vi "Detect Freeze.vi"(8 "error in (no error)":errorcluster, 11 "Running image Index":i32) -> (0 "error out":errorcluster)   [LabVIEW 2013]
doc: "Use this template to build a VI to use as a subVI."
uses:
  DB/DbEnum.ctl
  TypeDef/GreyLevelData.ctl
  DB/DisplayGFVEnum.ctl
  DB/DisplayDB.ctl
  <vilib>/vision/Image Controls.llb/IMAQ Image.ctl
  DB/ConfDB.ctl
  DB/ConfEnum.ctl
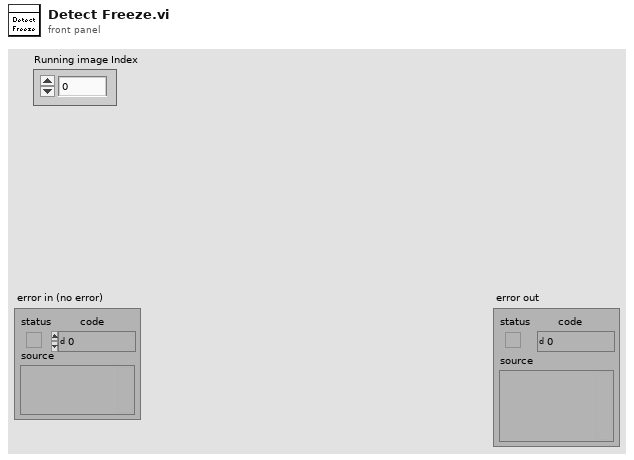
[diagram p1: front panel]
types:
  T1 = typedef "ConfEnum.ctl" = enum16{"Init", "GetConfDB", "Configure DB"}
  T2 = typedef "ConfDB.ctl" = cluster{"NumberOfImages":i32, "NoImages2SaveAroundFreeze":i32, "Path":path, "NameOfPartialFile":string, "StartIndex":i32, "NumberOfStdTol":i32, "Detla t (sec)":i32, "Number of images for baseline":i32, "Temperature File Name":string, "Score":dbl, "Index number of Files":i32[], "End Index":i32}
  T3 = cluster{"ImageIndexArray":u32[], "GreyLevelInBoundingBox":dbl[][], "GLDifference":dbl[][]}
  T4 = typedef "DbEnum.ctl" = enum16{"Init", "Insert Detection Result Data", "Insert Grey Level Result", "Insert Baseline Results", "Insert Freeze Analysis Results", "GetDropDB", "GetGreyLevelAndDiff", "GetGreyLevelatIndexTime", "GetDropletsBoundingBox"}
  T5 = typedef "DisplayDB.ctl" = cluster{"Image Ref":T6}
  T6 = typedef "IMAQ Image.ctl" = refnum<image>
  T7 = typedef "DisplayGFVEnum.ctl" = enum16{"Update Display", "Get Image Ref", "Insert Image Ref to Display", "Init Display"}
  T8 = typedef "GreyLevelData.ctl" = cluster{"Grey Level":dbl[], "Grey level diff":dbl[], "ImageIndex":u32, "Drop Index":u32}
  T9 = typedef "FreezePointData.ctl" = cluster{"Freeze YesNo":cluster{"Freeze Grey Diff value":dbl, "Freeze Index":u32, "Freeze Point Found":bool}[], "Rel Time":u32[]}
  T10 = cluster{"DropletBaseline":dbl[], "DropletBaselineSTD":dbl[]}
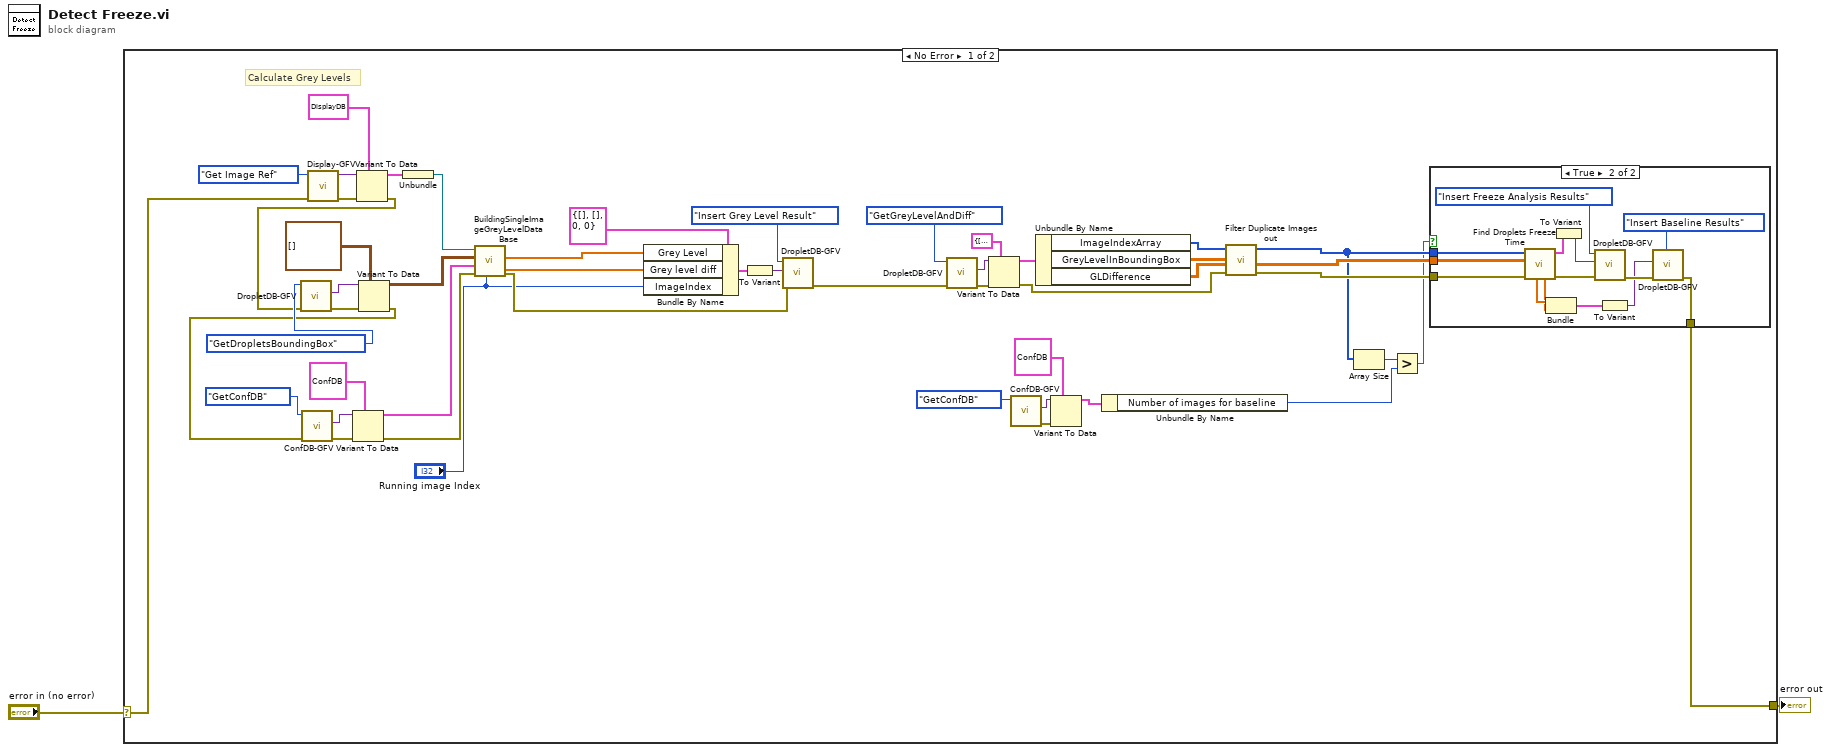
[diagram p0: block diagram]
diagram:
  n1 = case shown="No Error" "error in (no error)" {
    selector: "error in (no error)" -> [w33 w68]
    tunnel: [w12 w68] -> w1
    frame No Error {
      # "Calculate Grey Levels"
      n2 = call "Display-GFV.vi"("error in (no error)"=w33, 11:DisplayGFVEnum."Get Image Ref") -> ("error out"=w49:errorcluster, "Data out"=w48:variant)  [unwired: 7 in, 1 out]
      n3 = Variant To Data(error in=w49, type=T5 {"Image Ref"=refnum} ("Display Cluster"), Variant=w48) -> (data=w50:T5, error out=w32:errorcluster)
      n4 = call "DropletDB-GFV.vi"("error in (no error)"=w32, "Command In"=DbEnum."GetDropletsBoundingBox") -> ("error out"=w39:errorcluster, "Data out"=w40:variant)  [unwired: 8 in]
      n5 = Variant To Data(error in=w39, type=cluster{"x":sgl, "y":sgl}[][] [] ("Bounding Box"), Variant=w40) -> (data=w52:cluster{"x":sgl, "y":sgl}[][], error out=w31:errorcluster)
      n6 = call "ConfDB-GFV.vi"("error in (no error)"=w31, "Command In"=ConfEnum."GetConfDB") -> ("error out"=w35:errorcluster, "Data out"=w36:variant)  [unwired: 8 in]
      n7 = Variant To Data(error in=w35, type=T2 {"NumberOfImages"=0, "NoImages2SaveAroundFreeze"=0, "Path"=path "", "NameOfPartialFile"="", "StartIndex"=0, "NumberOfStdTol"=0, "Detla t (sec)"=0, "Number of images for baseline"=0, "Temperature File Name"="", "Score"=0.0, "Index number of Files"=[], "End Index"=0} ("ConfDB"), Variant=w36) -> (data=w26:T2, error out=w30:errorcluster)
      n8 = Unbundle(w50) -> ("Image Ref"=w51:T6)
      n9 = call "BuildingSingleImageGreyLevelDataBase.vi"("Running Index"="Running image Index", "error in (no error)"=w30, "ConfDB"=w26, "Droplet Bounding Box"=w52, "Image Ref In"=w51) -> ("error out"=w27:errorcluster, "Difference in Grey Level"=w28:dbl[], "GreyLevelArray"=w29:dbl[])  [unwired: 4 in]
      n10 = Bundle By Name(cluster=T8 {"Grey Level"=[], "Grey level diff"=[], "ImageIndex"=0, "Drop Index"=0} ("Cluster"), "Grey Level"=w29, "Grey level diff"=w28, "ImageIndex"="Running image Index") -> (w44:T8)
      n11 = To Variant(anything=w44) -> (Variant=w43:variant)
      n12 = call "DropletDB-GFV.vi"("error in (no error)"=w27, "Data in"=w43, "Command In"=DbEnum."Insert Grey Level Result") -> ("error out"=w23:errorcluster)  [unwired: 7 in, 1 out]
      n13 = call "DropletDB-GFV.vi"("error in (no error)"=w23, "Command In"=DbEnum."GetGreyLevelAndDiff") -> ("error out"=w22:errorcluster, "Data out"=w21:variant)  [unwired: 8 in]
      n14 = Variant To Data(error in=w22, type=T3 {"ImageIndexArray"=[], "GreyLevelInBoundingBox"=[], "GLDifference"=[]} ("output cluster"), Variant=w21) -> (data=w19:T3, error out=w15:errorcluster)
      n15 = call "ConfDB-GFV.vi"("Command In"=ConfEnum."GetConfDB") -> ("error out"=w7:errorcluster, "Data out"=w8:variant)  [unwired: 9 in]
      n16 = Unbundle By Name(w19) -> ("ImageIndexArray"=w18:u32[], "GreyLevelInBoundingBox"=w17:dbl[][], "GLDifference"=w16:dbl[][])
      n17 = Variant To Data(error in=w7, type=T2 {"NumberOfImages"=0, "NoImages2SaveAroundFreeze"=0, "Path"=path "", "NameOfPartialFile"="", "StartIndex"=0, "NumberOfStdTol"=0, "Detla t (sec)"=2, "Number of images for baseline"=0, "Temperature File Name"="", "Score"=0.0, "Index number of Files"=[], "End Index"=0} ("ConfDB"), Variant=w8) -> (data=w5:T2)  [unwired: 1 out]
      n18 = Unbundle By Name(w5) -> ("Number of images for baseline"=w4:i32)
      n19 = call "Filter Duplicate Images out.vi"("Error In"=w15, "GreyLevel Drops and time Derivative in"=w16, "GreyLevel Drops and time in"=w17, "Rel Time (s) in"=w18) -> ("Error Out"=w13:errorcluster, "GreyLevel Drops and time Derivative out"=w14:dbl[][], "Rel Time (s) out"=w11:u32[])  [unwired: 4 in, 1 out]
      n20 = Array Size(array=w11) -> (size(s)=w10:i32)
      n21 = Greater?(x=w10, y=w4) -> (0:w3:bool)
      n22 = case shown="True" w3 {
        tunnel: w14 -> [_ w67]
        tunnel: w13 -> [w53 w66]
        tunnel: [w53 w55] -> w12
        tunnel: w11 -> [_ w54]
        frame False {
        }
        frame True {
          n23 = call "Find Droplets Freeze Time.vi"("Error In"=w66, "GreyLevel Drops and time Derivative in"=w67, "Rel Time Array"=w54) -> ("Error Out"=w58:errorcluster, "FreezeYesNo"=w65:T9, "DropletBaselineSTD"=w60:dbl[], "DropletBaseline"=w61:dbl[])  [unwired: 3 in, 2 out]
          n24 = Bundle("DropletBaseline"=w61, "DropletBaselineSTD"=w60) -> (w62:T10)  [unwired: 1 in]
          n25 = To Variant(anything=w65) -> (Variant=w64:variant)
          n26 = call "DropletDB-GFV.vi"("error in (no error)"=w58, "Data in"=w64, "Command In"=DbEnum."Insert Freeze Analysis Results") -> ("error out"=w57:errorcluster)  [unwired: 7 in, 1 out]
          n27 = To Variant(anything=w62) -> (Variant=w56:variant)
          n28 = call "DropletDB-GFV.vi"("error in (no error)"=w57, "Data in"=w56, "Command In"=DbEnum."Insert Baseline Results") -> ("error out"=w55:errorcluster)  [unwired: 7 in, 1 out]
        }
      }
    }
    frame Error {
    }
  }
  "error out" <- w1
